vi "Save_Text_Big_Array_to_Excel_.vi"(8 "error in (no error)":errorcluster, 9 "start Position":cluster{"row":i32, "column":i32}={"row"=2, "column"=0}, 10 "배열":string[][](array[string]), 11 "report in":refnum<class "NI_report.lvclass">) -> (0 "error out":errorcluster, 3 "report out":refnum<class "NI_report.lvclass">)   [LabVIEW 2015]
uses:
  <vilib>/Utility/NIReport.llb/NI_report.lvclass
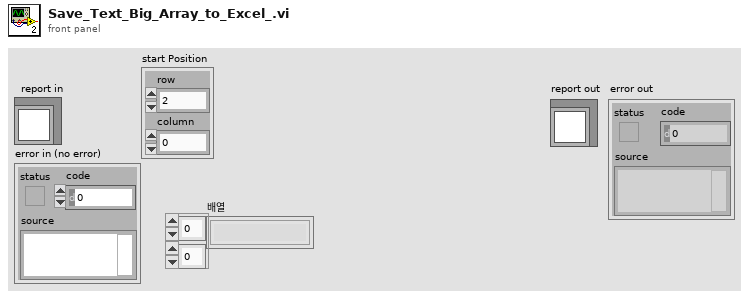
[diagram p1: front panel]
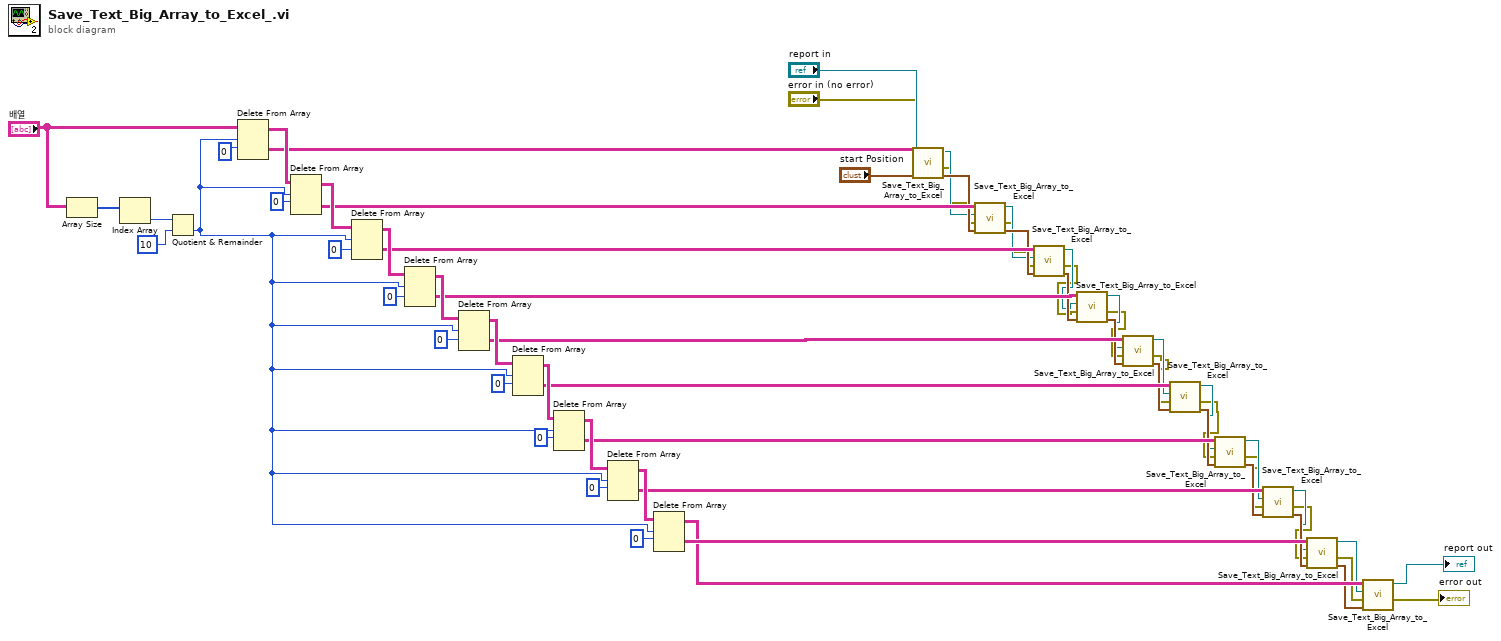
[diagram p0: block diagram]
diagram:
  n1 = Array Size(array="배열") -> (size(s)=w62:i32[])
  n2 = Index Array(array=w62) -> (element=w61:i32)  [unwired: 1 in]
  n3 = Quotient & Remainder(x=w61, y=10) -> (floor(x/y)=w43:i32)  [unwired: 1 out]
  n4 = Delete From Array(array="배열", length=w43, index (row)=0 ("인덱스 (행)")) -> (deleted portion=w42:string[][], array with subset deleted=w60:string[][])  [unwired: 1 in]
  n5 = Delete From Array(array=w60, length=w43, index (row)=0 ("인덱스 (행)")) -> (deleted portion=w41:string[][], array with subset deleted=w59:string[][])  [unwired: 1 in]
  n6 = Delete From Array(array=w59, length=w43, index (row)=0 ("인덱스 (행)")) -> (deleted portion=w39:string[][], array with subset deleted=w58:string[][])  [unwired: 1 in]
  n7 = Delete From Array(array=w58, length=w43, index (row)=0 ("인덱스 (행)")) -> (deleted portion=w37:string[][], array with subset deleted=w57:string[][])  [unwired: 1 in]
  n8 = Delete From Array(array=w57, length=w43, index (row)=0 ("인덱스 (행)")) -> (deleted portion=w35:string[][], array with subset deleted=w56:string[][])  [unwired: 1 in]
  n9 = Delete From Array(array=w56, length=w43, index (row)=0 ("인덱스 (행)")) -> (deleted portion=w33:string[][], array with subset deleted=w54:string[][])  [unwired: 1 in]
  n10 = Delete From Array(array=w54, length=w43, index (row)=0 ("인덱스 (행)")) -> (deleted portion=w31:string[][], array with subset deleted=w55:string[][])  [unwired: 1 in]
  n11 = Delete From Array(array=w55, length=w43, index (row)=0 ("인덱스 (행)")) -> (deleted portion=w29:string[][], array with subset deleted=w53:string[][])  [unwired: 1 in]
  n12 = Delete From Array(array=w53, length=w43, index (row)=0 ("인덱스 (행)")) -> (deleted portion=w27:string[][], array with subset deleted=w25:string[][])  [unwired: 1 in]
  n13 = call "Save_Text_Big_Array_to_Excel.vi"("start Position"="start Position", "error in (no error)"="error in (no error)", "report in"="report in", "배열"=w42) -> ("Next position"=w40:cluster{"row":i32, "column":i32}, "error out"=w14:errorcluster, "report out"=w23:refnum<class "NI_report.lvclass">)  [unwired: 5 in]
  n14 = call "Save_Text_Big_Array_to_Excel.vi"("start Position"=w40, "error in (no error)"=w14, "report in"=w23, "배열"=w41) -> ("Next position"=w38:cluster{"row":i32, "column":i32}, "error out"=w13:errorcluster, "report out"=w22:refnum<class "NI_report.lvclass">)  [unwired: 5 in]
  n15 = call "Save_Text_Big_Array_to_Excel.vi"("start Position"=w38, "error in (no error)"=w13, "report in"=w22, "배열"=w39) -> ("Next position"=w36:cluster{"row":i32, "column":i32}, "error out"=w12:errorcluster, "report out"=w21:refnum<class "NI_report.lvclass">)  [unwired: 5 in]
  n16 = call "Save_Text_Big_Array_to_Excel.vi"("start Position"=w36, "error in (no error)"=w12, "report in"=w21, "배열"=w37) -> ("Next position"=w34:cluster{"row":i32, "column":i32}, "error out"=w11:errorcluster, "report out"=w20:refnum<class "NI_report.lvclass">)  [unwired: 5 in]
  n17 = call "Save_Text_Big_Array_to_Excel.vi"("start Position"=w34, "error in (no error)"=w11, "report in"=w20, "배열"=w35) -> ("Next position"=w32:cluster{"row":i32, "column":i32}, "error out"=w10:errorcluster, "report out"=w19:refnum<class "NI_report.lvclass">)  [unwired: 5 in]
  n18 = call "Save_Text_Big_Array_to_Excel.vi"("start Position"=w32, "error in (no error)"=w10, "report in"=w19, "배열"=w33) -> ("Next position"=w30:cluster{"row":i32, "column":i32}, "error out"=w9:errorcluster, "report out"=w18:refnum<class "NI_report.lvclass">)  [unwired: 5 in]
  n19 = call "Save_Text_Big_Array_to_Excel.vi"("start Position"=w30, "error in (no error)"=w9, "report in"=w18, "배열"=w31) -> ("Next position"=w28:cluster{"row":i32, "column":i32}, "error out"=w8:errorcluster, "report out"=w17:refnum<class "NI_report.lvclass">)  [unwired: 5 in]
  n20 = call "Save_Text_Big_Array_to_Excel.vi"("start Position"=w28, "error in (no error)"=w8, "report in"=w17, "배열"=w29) -> ("Next position"=w26:cluster{"row":i32, "column":i32}, "error out"=w7:errorcluster, "report out"=w16:refnum<class "NI_report.lvclass">)  [unwired: 5 in]
  n21 = call "Save_Text_Big_Array_to_Excel.vi"("start Position"=w26, "error in (no error)"=w7, "report in"=w16, "배열"=w27) -> ("Next position"=w24:cluster{"row":i32, "column":i32}, "error out"=w6:errorcluster, "report out"=w15:refnum<class "NI_report.lvclass">)  [unwired: 5 in]
  n22 = call "Save_Text_Big_Array_to_Excel.vi"("start Position"=w24, "error in (no error)"=w6, "report in"=w15, "배열"=w25) -> ("error out"=→"error out":errorcluster, "report out"=→"report out":refnum<class "NI_report.lvclass">)  [unwired: 5 in, 1 out]
